vi "PH_TKTDS-30xx.Fetch Waveform.vi"(0 "i ref in":refnum<vi>, 2 "Waveform to fetch":T2={"Source"="CH1", "Waveform Start"=1, "Waveform End"=10000}, 5 "error IO":errorcluster) -> (14 "i ref out":refnum<vi>, 19 "error out":errorcluster)   [LabVIEW 2014, in "PH_TKTDS-30xx.lvlib"]
doc: "If the connection is established, the waveform to fetched is fetched and written to own attributes as well as the errors."
uses:
  PH_TKTDS-30xx.lvlib
  PH_TKTDS-30xx.Waveform to fetch.ctl
  PH_TKTDS-30xx.fetched Waveform.ctl
  instr.lib/TKDS3032-PHELIX/tktds3032-PHELIX - Driver np.lvlib
panel:
  in  "Ch Config":T1={"Source"="CH1", "Actual Points"=0, "Initial X"=0.0, "X Increment"=1.0, "Waveform Array"=[]} {"Waveform Array" format="%.2f"; "X Increment" format="%.2e"; "Initial X" format="%.2e"}
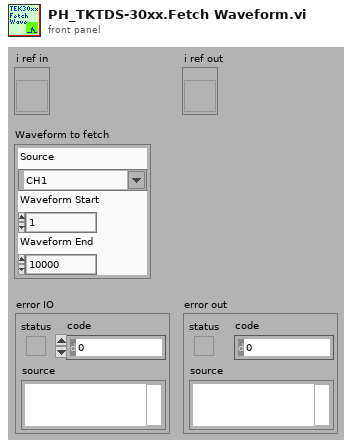
[diagram p1: front panel]
types:
  T1 = typedef "PH_TKTDS-30xx.lvlib/PH_TKTDS-30xx.fetched Waveform.ctl" = cluster{"Source":string, "Actual Points":u32, "Initial X":dbl, "X Increment":dbl, "Waveform Array":dbl[]}
  T2 = typedef "PH_TKTDS-30xx.lvlib/PH_TKTDS-30xx.Waveform to fetch.ctl" = cluster{"Source":string, "Waveform Start":i32, "Waveform End":i32}
  T3 = typedef "PH_TKTDS-30xx.lvlib/PH_TKTDS-30xx.i attribute.ctl" = cluster{"Default VISA Resource":string, "VISA Resource Name":refnum<visa-resource-name>, "Revision":cluster{"Instrument Driver":string, "Instrument Firmware":string}, "Selftest":cluster{"Result":u32, "Message":string}, "Channels":T4[], "Trigger Configuration":T5, "Acquisition Configuration":T6, "Fetched Waveforms":T1[], "GUI Refs":T7, "GUI Refs Channels":refnum<vi>[], "State":T8, "Error Message":string, "Allow Prdc Loop?":bool}
  T4 = typedef "PH_TKTDS-30xx.lvlib/PH_TKTDS-30xx.Channel Config.ctl" = cluster{"Channel Name":string, "Input Impedance":string, "Max Input Frequency":string, "Vertical Coupling":i32, "Channel Enabled":bool, "Probe Attenuation":dbl, "Vertical Range":dbl, "Vertical Offset":dbl}
  T5 = typedef "PH_TKTDS-30xx.lvlib/PH_TKTDS-30xx.Trigger Config.ctl" = cluster{"Source":string, "Slope":i32, "Level [V]":dbl}
  T6 = typedef "PH_TKTDS-30xx.lvlib/PH_TKTDS-30xx.Acquisition Config.ctl" = cluster{"Time base":dbl, "Record Length":u16, "Start Time":dbl, "Type":i32, "Continuous":bool}
  T7 = typedef "PH_TKTDS-30xx.lvlib/PH_TKTDS-30xx.GUI Refs.ctl" = cluster{"Trigger":refnum<vi>, "Acquisition":refnum<vi>, "Graph":refnum<vi>, "State":refnum<vi>, "Delete":refnum<vi>, "Channel to be positioned":refnum<vi>, "Postion":refnum<vi>, "Display Intensity":refnum<vi>, "VISA Resource":refnum<vi>}
  T8 = typedef "PH_StatusHandler.lvlib/PH_StatusHandler.Status.ctl" = i16
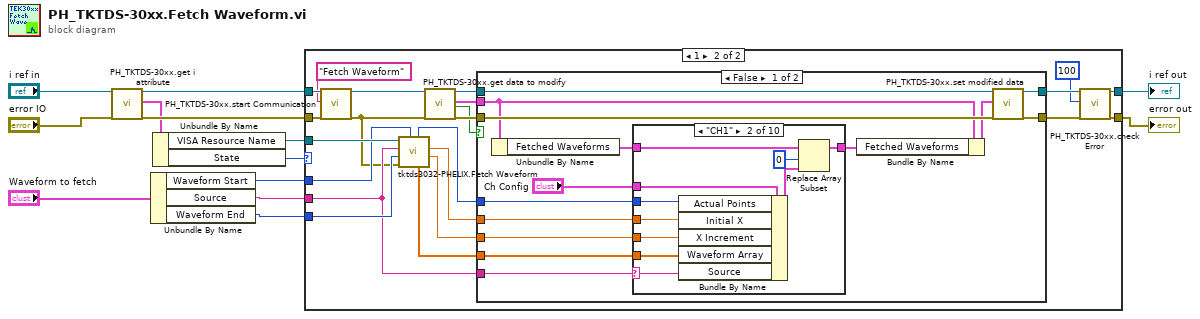
[diagram p0: block diagram]
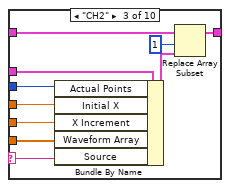
[diagram p4: hidden frame]
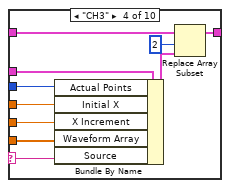
[diagram p5: hidden frame]
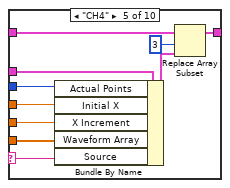
[diagram p6: hidden frame]
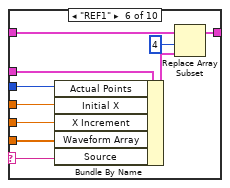
[diagram p7: hidden frame]
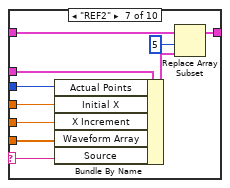
[diagram p8: hidden frame]
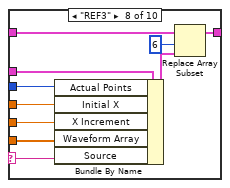
[diagram p9: hidden frame]
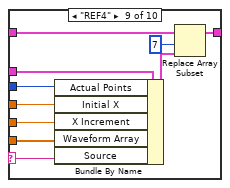
[diagram p10: hidden frame]
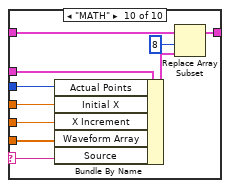
[diagram p11: hidden frame]
diagram:
  n1 = call "PH_TKTDS-30xx.get i attribute.vi"("i ref in"="i ref in", "error in (no error)"="error IO") -> ("i ref out"=w8:refnum<vi>, "i attribute"=w10:T3, "error out"=w12:errorcluster)  [unwired: 15 in]
  n2 = Unbundle By Name("Waveform to fetch") -> ("Waveform Start"=w1:i32, "Source"=w5:string, "Waveform End"=w4:i32)
  n3 = Unbundle By Name(w10) -> ("VISA Resource Name"=w11:refnum<visa-resource-name>, "State"=w3:T8)
  n4 = case shown="1" w3 {
    tunnel: w8 -> [w15 w22]
    tunnel: w11 -> [_ w37]
    tunnel: [w14 w20] -> w6
    tunnel: w12 -> [w14 w36]
    tunnel: [w15 w18] -> w13
    tunnel: w5 -> [_ w28]
    tunnel: w4 -> [_ w34]
    tunnel: w1 -> [_ w35]
    frame Default {
    }
    frame 1 {
      n5 = call "PH_TKTDS-30xx.start Communication.vi"("i ref in"=w22, "Action"="Fetch Waveform", "error in"=w36) -> ("i ref out"=w21:refnum<vi>, "error out"=w23:errorcluster)  [unwired: 15 in]
      n6 = call "tktds3032-PHELIX.Fetch Waveform.vi"("Waveform Start (1)"=w35, "error in (no error)"=w23, "Waveform End (10000)"=w34, "Source (Channel 1)"=w28, "VISA Resource Name"=w37) -> ("X Increment"=w25:dbl, "Initial X"=w26:dbl, "Waveform Array"=w24:dbl[], "Actual Points"=w27:u32)  [unwired: 1 in, 2 out]
      n7 = call "PH_TKTDS-30xx.get data to modify.vi"("i ref in"=w21, "error in (no error)"=w23) -> ("i ref out"=w33:refnum<vi>, "i attribute"=w30:T3, "timed out"=w29:bool, "error out"=w32:errorcluster)  [unwired: 14 in]
      n8 = case shown="False" w29 {
        tunnel: [w51 w143] -> w31
        tunnel: w32 -> [w50 w143]
        tunnel: w33 -> [w49 w144]
        tunnel: [w48 w144] -> w19
        tunnel: w30 -> [w46 _]
        tunnel: w28 -> [w45 _]
        tunnel: w27 -> [w42 _]
        tunnel: w24 -> [w41 _]
        tunnel: w25 -> [w40 _]
        tunnel: w26 -> [w38 _]
        frame False {
          n9 = Unbundle By Name(w46) -> ("Fetched Waveforms"=w43:T1[])
          n10 = case shown="\"CH1\"" w45 {
            selector: w45 -> [_ w53 w63 w73 w83 w93 w103 w113 w123 w133]
            tunnel: [w52 w61 w71 w81 w91 w101 w111 w121 w131 w141] -> w44
            tunnel: w43 -> [w52 w62 w72 w82 w92 w102 w112 w122 w132 w142]
            tunnel: w42 -> [_ w58 w68 w78 w88 w98 w108 w118 w128 w138]
            tunnel: w38 -> [_ w57 w67 w77 w87 w97 w107 w117 w127 w137]
            tunnel: w41 -> [_ w54 w64 w74 w84 w94 w104 w114 w124 w134]
            tunnel: w40 -> [_ w55 w65 w75 w85 w95 w105 w115 w125 w135]
            tunnel: "Ch Config" -> [_ w56 w66 w76 w86 w96 w106 w116 w126 w136]
            frame Default {
            }
            frame "CH1" {
              n11 = Bundle By Name(cluster=w56, "Actual Points"=w58, "Initial X"=w57, "X Increment"=w55, "Waveform Array"=w54, "Source"=w53) -> (w59:T1)
              n12 = Replace Array Subset(array=w62, new element=w59, index=0) -> (w61:T1[])
            }
            frame "CH2" {
              n13 = Bundle By Name(cluster=w66, "Actual Points"=w68, "Initial X"=w67, "X Increment"=w65, "Waveform Array"=w64, "Source"=w63) -> (w69:T1)
              n14 = Replace Array Subset(array=w72, new element=w69, index=1) -> (w71:T1[])
            }
            frame "CH3" {
              n15 = Bundle By Name(cluster=w76, "Actual Points"=w78, "Initial X"=w77, "X Increment"=w75, "Waveform Array"=w74, "Source"=w73) -> (w79:T1)
              n16 = Replace Array Subset(array=w82, new element=w79, index=2) -> (w81:T1[])
            }
            frame "CH4" {
              n17 = Bundle By Name(cluster=w86, "Actual Points"=w88, "Initial X"=w87, "X Increment"=w85, "Waveform Array"=w84, "Source"=w83) -> (w89:T1)
              n18 = Replace Array Subset(array=w92, new element=w89, index=3) -> (w91:T1[])
            }
            frame "REF1" {
              n19 = Bundle By Name(cluster=w96, "Actual Points"=w98, "Initial X"=w97, "X Increment"=w95, "Waveform Array"=w94, "Source"=w93) -> (w99:T1)
              n20 = Replace Array Subset(array=w102, new element=w99, index=4) -> (w101:T1[])
            }
            frame "REF2" {
              n21 = Bundle By Name(cluster=w106, "Actual Points"=w108, "Initial X"=w107, "X Increment"=w105, "Waveform Array"=w104, "Source"=w103) -> (w109:T1)
              n22 = Replace Array Subset(array=w112, new element=w109, index=5) -> (w111:T1[])
            }
            frame "REF3" {
              n23 = Bundle By Name(cluster=w116, "Actual Points"=w118, "Initial X"=w117, "X Increment"=w115, "Waveform Array"=w114, "Source"=w113) -> (w119:T1)
              n24 = Replace Array Subset(array=w122, new element=w119, index=6) -> (w121:T1[])
            }
            frame "REF4" {
              n25 = Bundle By Name(cluster=w126, "Actual Points"=w128, "Initial X"=w127, "X Increment"=w125, "Waveform Array"=w124, "Source"=w123) -> (w129:T1)
              n26 = Replace Array Subset(array=w132, new element=w129, index=7) -> (w131:T1[])
            }
            frame "MATH" {
              n27 = Bundle By Name(cluster=w136, "Actual Points"=w138, "Initial X"=w137, "X Increment"=w135, "Waveform Array"=w134, "Source"=w133) -> (w139:T1)
              n28 = Replace Array Subset(array=w142, new element=w139, index=8) -> (w141:T1[])
            }
          }
          n29 = Bundle By Name(cluster=w46, "Fetched Waveforms"=w44) -> (w47:T3)
          n30 = call "PH_TKTDS-30xx.set modified data.vi"("i ref in"=w49, "i attribute"=w47, "error in (no error)"=w50) -> ("i ref out"=w48:refnum<vi>, "error out"=w51:errorcluster)  [unwired: 15 in]
        }
        frame True {
        }
      }
      n31 = call "PH_TKTDS-30xx.check Error.vi"("i ref in"=w19, "Waiting Time [ms]"=u32 100, "error in"=w31) -> ("i ref out"=w18:refnum<vi>, "error out"=w20:errorcluster)  [unwired: 15 in]
    }
  }
  "i ref out" <- w13
  "error out" <- w6
